vi "Write RDS message Time Stamp.vi"(8 "error in (no error)":errorcluster, 10 "Time Stamp":timestamp, 11 "RDS Message in":refnum<class "RDS Message.lvclass">) -> (0 "error out":errorcluster, 3 "RDS Message out":refnum<class "RDS Message.lvclass">)   [LabVIEW 2015, in "RDS Child Messages.lvlib" / "RDS Message.lvclass"]
uses:
  RDS Message.lvclass
  RDS Message.lvclass/RDS Message.ctl
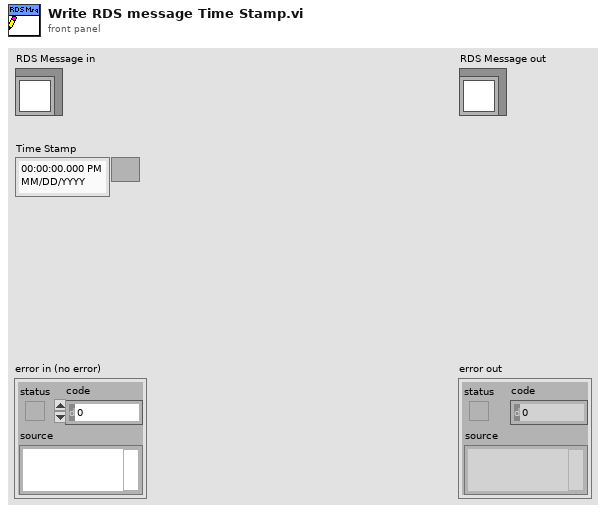
[diagram p1: front panel]
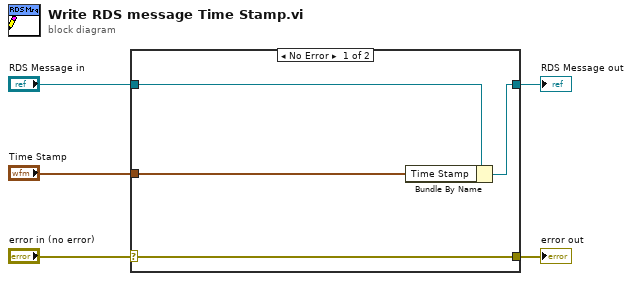
[diagram p0: block diagram]
diagram:
  n1 = case shown="No Error" "error in (no error)" {
    selector: "error in (no error)" -> [w9 w10]
    tunnel: [w9 w10] -> w4
    tunnel: [w7 w11] -> w2
    tunnel: "RDS Message in" -> [w8 w11]
    tunnel: "Time Stamp" -> [w6 _]
    frame No Error {
      n2 = Bundle By Name(cluster=w8, "Time Stamp"=w6) -> (w7:refnum<class "RDS Message.lvclass">)
    }
    frame Error {
    }
  }
  "error out" <- w4
  "RDS Message out" <- w2
